vi "data_input.vi"() -> ()   [LabVIEW 2026]
uses:
  <vilib>/DAQmx/read.llb/DAQmx Read.vi
  <vilib>/DAQmx/read.llb/DAQmx Read (Analog 1D Wfm NChan NSamp).vi
  <vilib>/DAQmx/miscellaneous.llb/DAQmx Fill In Error Info.vi
panel:
  out "mean":dbl
  in  "stop":bool
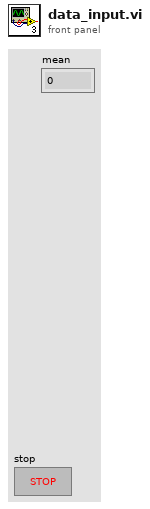
[diagram p1: front panel]
types:
  T1 = enum16{"open", "open or create", "create or replace", "create", "open (read only)"}
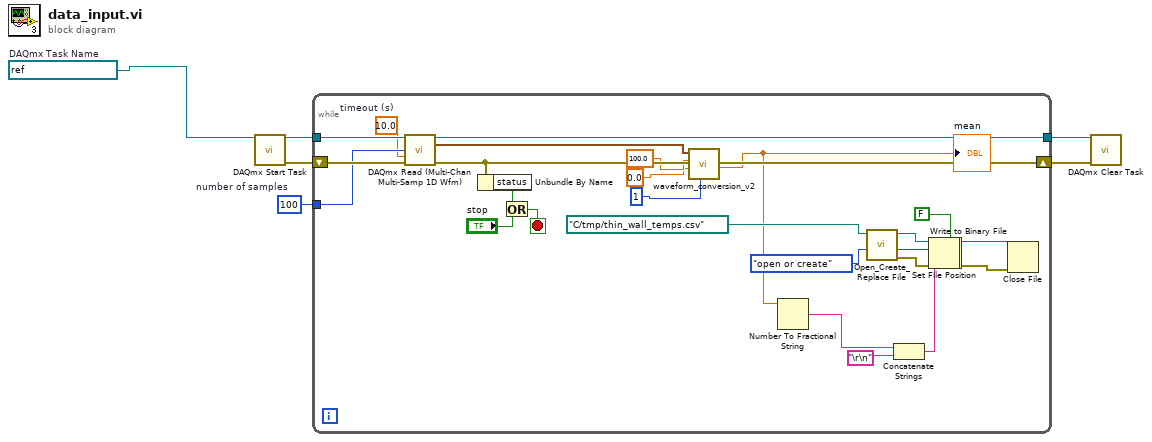
[diagram p0: block diagram]
diagram:
  w1 = refnum<k21> "MyVoltageTask"  # DAQmx Task Name
  w4 = 100  # number of samples
  n1 = call <vilib>:"DAQmx Start Task.vi"("task/channels in"=w1) -> ("task out"=w6:refnum<k21>, "error out"=w5:errorcluster)  [unwired: 13 in]
  n2 = while {
    tunnel: w6 -> [w33]
    tunnel: w4 -> [w30]
    tunnel: [w31] -> w2
    shift-right: [w28] -> w3
    shift-left: w5 -> [w32]
    stop <- w27 stop-if-true
    w25 = 10.0  # timeout (s)
    n3 = call-poly "DAQmx Read (Multi-Chan Multi-Samp 1D Wfm).vi"("task/channels in"=w33, "number of samples per channel"=w30, "timeout"=w25, "error in"=w32) -> ("task out"=w31:refnum<k21>, "data"=w22:waveform(dbl)[], "error out"=w28:errorcluster)  [unwired: 9 in]
    n4 = Unbundle By Name(w28) -> ("status"=w29:bool)
    n5 = Or(x=w29, y="stop") -> (x .or. y?=w27:bool)
    n6 = call "waveform_conversion_v2.vi"("sample length"=1, "y"=0.0, "y 2"=100.0 ("y"), "data"=w22) -> ("mean"=w7:dbl)  [unwired: 7 in]
    "mean" <- w7
    n7 = Number To Fractional String(number=w7) -> (F-format string=w8:string)  [unwired: 3 in]
    n8 = call <vilib>:"Open_Create_Replace File.vi"("function (open:0)"=T1."open or create", "file path"=path "C:/tmp/thin_wall_temps.csv" ("file (use dialog)")) -> ("error out"=w11:errorcluster, "file size (bytes)"=w13:i32, "refnum"=w12:refnum<file>)  [unwired: 6 in, 1 out]
    n9 = Concatenate Strings(w8, "\r\n") -> (w17:string)
    n10 = Set File Position(offset (in bytes) (0)=w13, refnum=w12, error in=w11) -> (refnum out=w18:refnum<file>, error out=w19:errorcluster)  [unwired: 1 in]
    n11 = Write to Binary File(file (use dialog)=w18, data=w17, error in=w19, 5:FALSE ("prepend array or string size? (T)")) -> (refnum out=w15:refnum<file>, error out=w14:errorcluster)  [unwired: 2 in, 1 out]
    n12 = Close File(refnum=w15, error in=w14) -> ()  [unwired: 2 out]
  }
  n13 = call <vilib>:"DAQmx Clear Task.vi"("task in"=w2, "error in"=w3) -> ()  [unwired: 13 in, 1 out]
